vi "DT_Find First Triangulation.vi"(7 "length":i32, 8 "cur point":i32, 11 "Points In":cluster{"x":dbl, "y":dbl, "index":i32}[](array[cluster])) -> (0 "next point":i32, 1 "next triangle":i32, 2 "Triangles":i32[][](array[numeric]), 3 "Points Out":cluster{"x":dbl, "y":dbl, "index":i32}[](array[cluster]))   [LabVIEW 2017, in "NI_AAL_Geometry.lvlib"]
uses:
  <vilib>/Analysis/NI_AAL_Geometry.lvlib
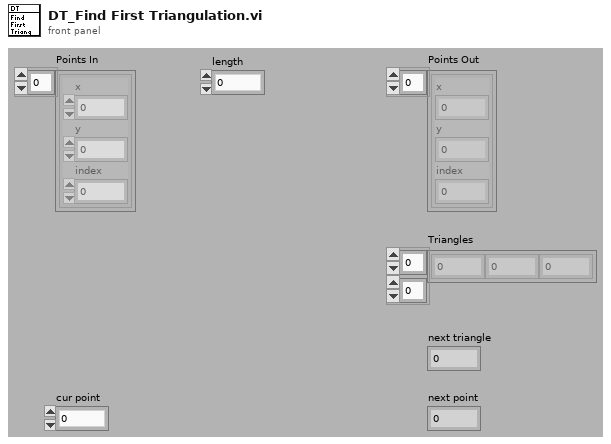
[diagram p1: front panel]
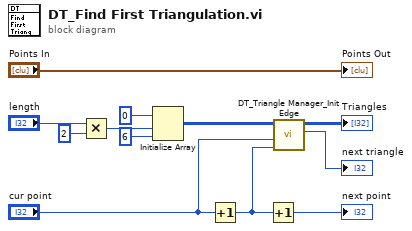
[diagram p0: block diagram]
diagram:
  n1 = Multiply(x="length", y=2) -> (x*y=w11:i32)
  n2 = Initialize Array(0 ("y"), w11, 6 ("dimension size")) -> (w7:i32[][])
  n3 = Increment(x="cur point") -> (x+1=w3:i32)
  n4 = Increment(x=w3) -> (x+1=→"next point":i32)
  n5 = call <vilib>:"DT_Triangle Manager_Init Edge.vi"("right point"=w3, "left point"="cur point", "Triangles In"=w7) -> ("next triangle out"=→"next triangle":i32, "Triangles Out"=→"Triangles":i32[][])  [unwired: 1 in, 6 out]
  "Points Out" <- "Points In"
